vi "Two 32-bit Port Digital Input.vi"(2 "Two 32-bit DI Ports":T1={"32-bit DI Port 0"="Chassis1/Mod4/DI7:0", "32-bit DI Port 1"="Chassis1/Mod4/DI7:0"}) -> (7 "Packet":u64)   [LabVIEW 2009]
uses:
  <vilib>/eio/EIONode/EIONode.xnode
  <vilib>/rvi/eio/nirviEIOImplementation/nirviEIOImplementation.xnode
  <vilib>/rvi/eio/common/nirviEmuTemplateMethod_noerrors.vi
  <vilib>/rvi/eio/common/nirviEmuClasses.ctl
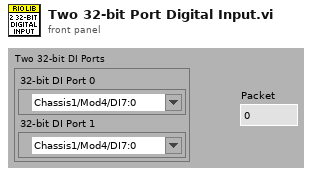
[diagram p1: front panel]
types:
  T1 = cluster{"32-bit DI Port 0":refnum<k21>, "32-bit DI Port 1":refnum<k21>}
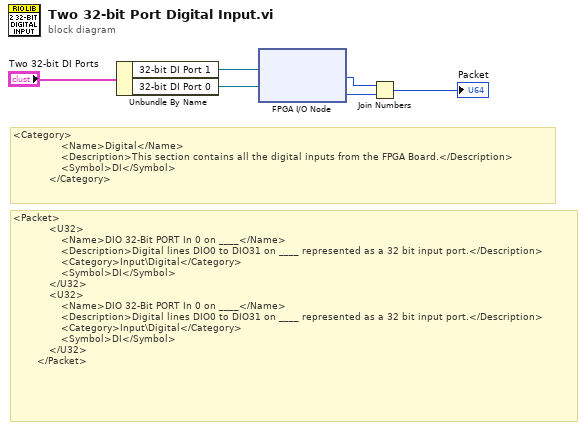
[diagram p0: block diagram]
diagram:
  # "<Packet>\n            <U32>\n                <Name>DIO 32-Bit PORT In 0 on ____</Name>\n                <Description>Digital lines DIO0 to DIO31 on ____ represented as a 32 bit input port.</Description>\n                <Category>Input\\Digital</Category>\n                <Symbol>DI</Symbol>\n            </U32>\n            <U32>\n                <Name>DIO 32-Bit PORT In 0 on ____</Name>\n                <Description>Digital lines DIO0 to DIO31 on ____ represented as a 32 bit input port.</Description>\n                <Category>Input\\Digital</Category>\n                <Symbol>DI</Symbol>\n            </U32>\n        </Packet>"
  # "<Category>\n                <Name>Digital</Name>\n                <Description>This section contains all the digital inputs from the FPGA Board.</Description>\n                <Symbol>DI</Symbol>\n            </Category>"
  n1 = Unbundle By Name("Two 32-bit DI Ports") -> ("32-bit DI Port 1"=w2:refnum<k21>, "32-bit DI Port 0"=w3:refnum<k21>)
  n2 = xnode "FPGA I/O Node"("FPGA I/O In"=w2, "FPGA I/O In"=w3) -> ("I/O Item"=w1:u32, "I/O Item"=w6:u32)  [unwired: 2 out]
  n3 = Join Numbers(hi=w1, lo=w6) -> ((hi.lo)=→"Packet":u64)
